vi "Thermometer Reading with Write to text file with path control.vi"() -> ()   [LabVIEW 2020]
panel:
  in  "Path":path
  out "Waveform Chart":dbl(graph)
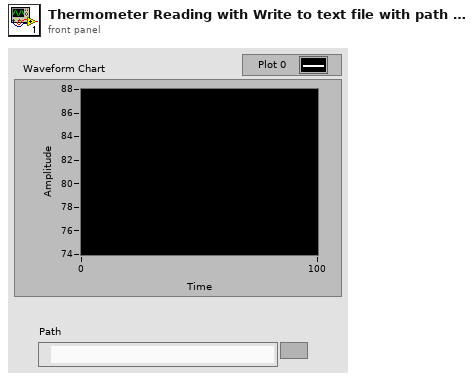
[diagram p1: front panel]
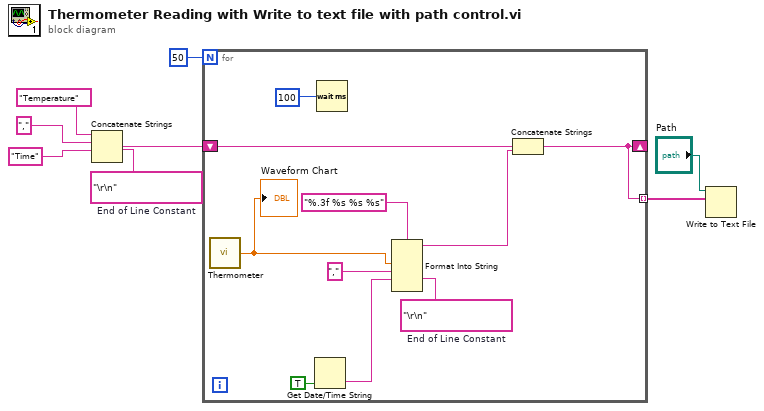
[diagram p0: block diagram]
diagram:
  w4 = "\r\n"  # End of Line Constant
  n1 = Concatenate Strings "Concatenate Strings"("Temperature" ("string"), "," ("string"), "Time" ("string"), w4) -> (w3:string)
  n2 = for {
    N: 50 -> [_]
    shift-right: [w9] -> _
    shift-left: w3 -> [w12]
    tunnel: [w9] -> w2 mode=indexing
    w14 = "\r\n"  # End of Line Constant
    n3 = call "Thermometer.vi"() -> ("Temperature (deg F)"=w10:dbl)  [unwired: 1 in]
    "Waveform Chart" <- w10
    n4 = Get Date/Time String(want seconds? (F)=TRUE) -> (time string=w16:string)  [unwired: 2 in, 1 out]
    n5 = Wait (ms)(milliseconds to wait=u32 100 ("millisecond timer value")) -> ()  [unwired: 1 out]
    n6 = Format Into String "Format Into String"(format string="%.3f %s %s %s", w10, "," ("input 2"), w16, w14) -> (resulting string=w13:string)  [unwired: 2 in, 1 out]
    n7 = Concatenate Strings "Concatenate Strings"(w12, w13) -> (w9:string)
  }
  n8 = Write to Text File(file (use dialog)="Path", text=w2) -> ()  [unwired: 2 in, 3 out]
